vi "WaitForSnapshot.vi"(4 "snapshotWaitMode":T1, 6 "context":string, 8 "error in (no error)":errorcluster, 9 "timeout_ms":i32, 10 "targetID":string, 11 "snapshotNotifier":refnum<notifier>) -> (0 "error out":errorcluster, 3 "snapshot":T2={"globalThreshold"=enum."INFO", "appenderEnqueuers"=[]})   [LabVIEW 2026, in "Lumberjack.lvlib" / "Logger.lvclass"]
doc: "Blocks until the manager's published Snapshot satisfies the selected condition, or the timeout expires; makes control-plane operations synchronous without sleeps. SnapshotWaitMode selects the condition: AnySnapshot (any Snapshot received = manager readiness, used by Initialize), IDPresent (an appender with targetID appears = registration confirmed, used by RegisterAppender), IDAbsent (no appender with targetID remains = unregistration confirmed, or the id was never present, used by UnregisterAppender). Uses a deadline computed once (deadline = start + timeout), each wait consuming the remaining time, so the total wait is bounded. Outputs a valid Snapshot only on the success path; on timeout returns error 5030 with the caller context. Control plane; not on the hot path."
uses:
  Logger.lvclass
  TypeDefs/Snapshot.ctl
  TypeDefs/Severity.ctl
  <vilib>/ActorFramework/Message Enqueuer/Message Enqueuer.lvclass
  TypeDefs/SnapshotWaitMode.ctl
  Logger.lvclass/Logger.ctl
  Lumberjack.lvlib
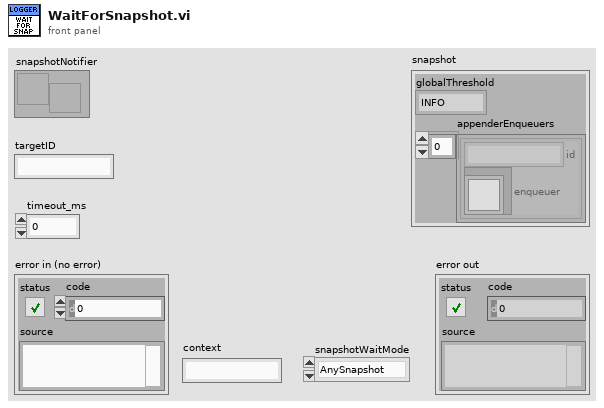
[diagram p1: front panel]
types:
  T1 = typedef "Lumberjack.lvlib/SnapshotWaitMode.ctl" = enum16{"AnySnapshot", "IDPresent", "IDAbsent"}
  T2 = typedef "Lumberjack.lvlib/Snapshot.ctl" = cluster{"globalThreshold":T3, "appenderEnqueuers":cluster{"id":string, "enqueuer":refnum<class "Message Enqueuer.lvclass">}[]}
  T3 = typedef "Lumberjack.lvlib/Severity.ctl" = enum16{"OFF", "FATAL", "ERROR", "WARN", "INFO", "DEBUG", "TRACE", "ALL"}
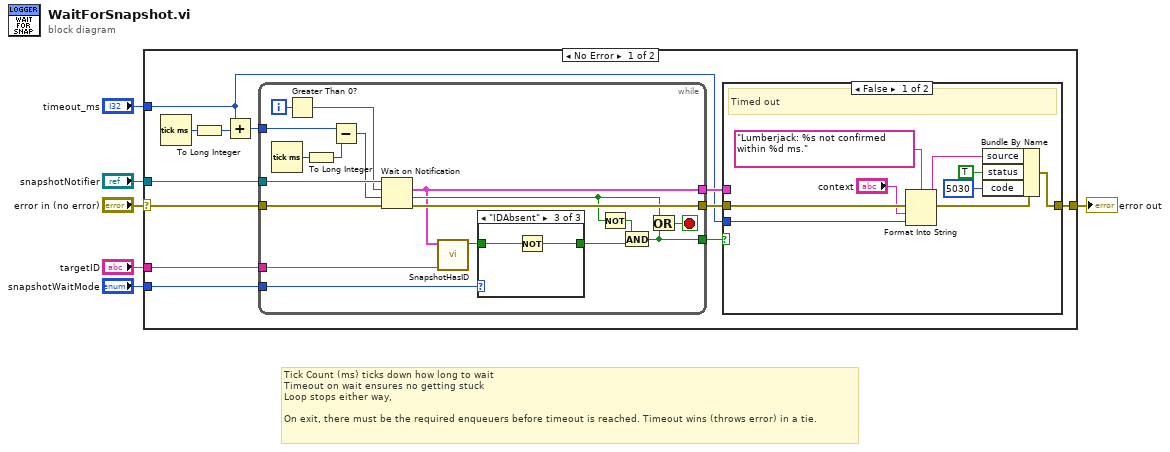
[diagram p0: block diagram]
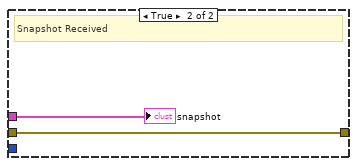
[diagram p2: hidden frame]
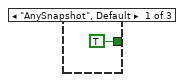
[diagram p3: hidden frame]
diagram:
  # "Tick Count (ms) ticks down how long to wait\nTimeout on wait ensures no getting stuck\nLoop stops either way, \n\nOn exit, there must be the required enqueuers before timeout is reached. Timeout wins (throws error) in a tie."
  n1 = case shown="No Error" "error in (no error)" {
    selector: "error in (no error)" -> [w16 w52]
    tunnel: "snapshotNotifier" -> [w18 _]
    tunnel: "targetID" -> [w17 _]
    tunnel: [w11 w52] -> w4
    tunnel: "timeout_ms" -> [w8 _]
    tunnel: "snapshotWaitMode" -> [w7 _]
    frame No Error {
      n2 = Tick Count (ms)() -> (millisecond timer value=w15:u32)
      n3 = To Long Integer(number=w15) -> (32bit integer=w14:i32)
      n4 = Add(x=w8, y=w14) -> (x+y=w13:i32)
      n5 = while {
        tunnel: w18 -> [w41]
        tunnel: w17 -> [w34]
        tunnel: w13 -> [w45]
        tunnel: [w33] -> w9
        tunnel: [w36] -> w10
        tunnel: w16 -> [w42]
        tunnel: [w47] -> w12
        tunnel: w7 -> [w32]
        i -> [w43]
        stop <- w38 stop-if-true
        n6 = Tick Count (ms)() -> (millisecond timer value=w46:u32)
        n7 = Greater Than 0?(x=w43) -> (x > 0?=w40:bool)
        n8 = To Long Integer(number=w46) -> (32bit integer=w44:i32)
        n9 = Subtract(x=w45, y=w44) -> (x-y=w39:i32)
        n10 = Wait on Notification(notifier=w41, ignore previous (F)=w40, timeout in ms (-1)=w39, error in (no error)=w42) -> (notification=w33:T2, timed out?=w35:bool, error out=w47:errorcluster)  [unwired: 1 out]
        n11 = call "SnapshotHasID.vi"("id"=w34, "Snapshot"=w33) -> ("found"=w31:bool)  [unwired: 9 in]
        n12 = case shown="\"IDAbsent\"" w32 {
          tunnel: w31 -> [_ w49 w51]
          tunnel: [TRUE ("found") w49 w50] -> w30
          frame "AnySnapshot", Default {
          }
          frame "IDPresent" {
          }
          frame "IDAbsent" {
            n13 = Not(x=w51) -> (.not. x?=w50:bool)
          }
        }
        n14 = Not(x=w35) -> (.not. x?=w37:bool)
        n15 = And(x=w37, y=w30) -> (x .and. y?=w36:bool)
        n16 = Or(x=w35, y=w36) -> (x .or. y?=w38:bool)
      }
      n17 = case shown="False" w10 {
        tunnel: w12 -> [w22 w28]
        tunnel: [w21 w28] -> w11
        tunnel: w9 -> [_ w29]
        tunnel: w8 -> [w19 _]
        frame False {
          # "Timed out"
          n18 = Format Into String(format string="Lumberjack: %s not confirmed within %d ms." ("source"), error in=w22, "context", w19) -> (resulting string=w24:string, error out=w25:errorcluster)  [unwired: 1 in]
          n19 = Bundle By Name(cluster=w25, "source"=w24, "status"=TRUE, "code"=5030) -> (w21:errorcluster)
        }
        frame True {
          # "Snapshot Received"
          "snapshot" <- w29
        }
      }
    }
    frame Error {
    }
  }
  "error out" <- w4
